vi "K2000_wait_get_array.vi"(2 "emergency exit":bool, 3 "samples":u64=4096, 4 "Readout parameters":T1(array[cluster])) -> (0 "requester status byte":i16, 1 "measures":sgl[][](array[numeric]))   [LabVIEW 2013]
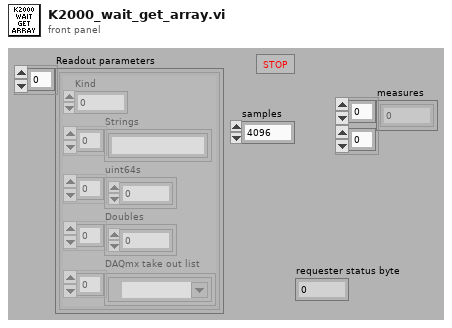
[diagram p1: front panel]
types:
  T1 = cluster{"Kind":u16, "Strings":string[], "uint64s":u64[], "Doubles":dbl[], "DAQmx take out list":refnum<k21>[]}[]
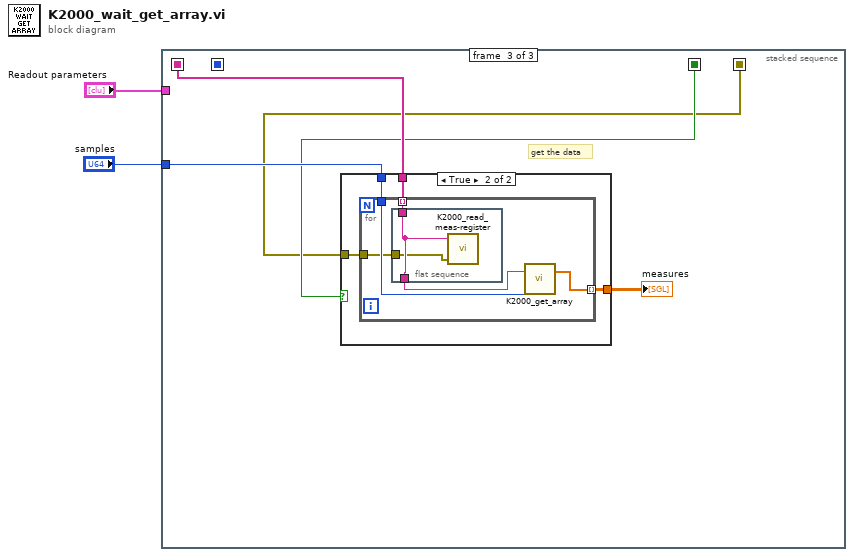
[diagram p0: block diagram]
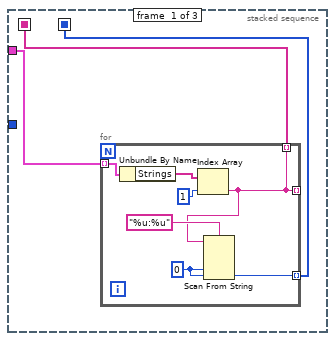
[diagram p2: hidden frame]
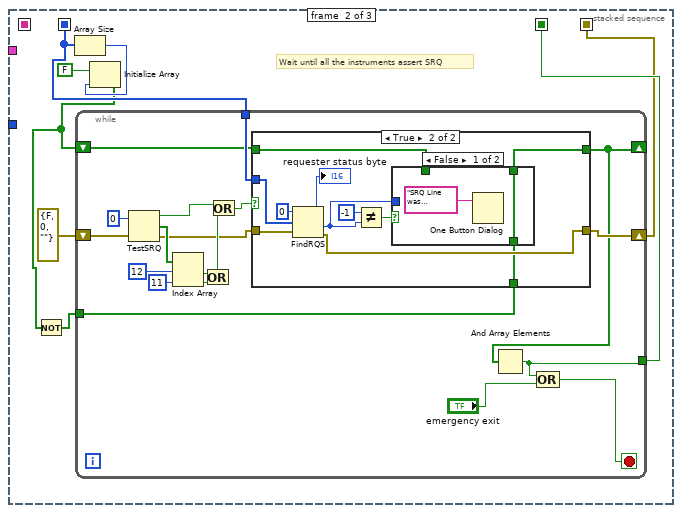
[diagram p3: hidden frame]
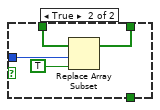
[diagram p5: hidden frame]
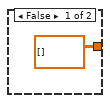
[diagram p6: hidden frame]
diagram:
  n1 = stacked-sequence {
    seq-local: [w4 _ _] -> [_ _ w62]
    seq-local: [w3 _ _] -> [_ w17 _]
    seq-local: [_ w14 _] -> [_ _ w60]
    seq-local: [_ w13 _] -> [_ _ w59]
    tunnel: "Readout parameters" -> [w5 _ _]
    tunnel: "samples" -> [_ _ w61]
    frame #0 {
      n2 = for {
        tunnel: w5 -> [w12] mode=indexing
        tunnel: [w6] -> _ mode=indexing
        tunnel: [w7] -> w3 mode=indexing
        tunnel: [w6] -> w4 mode=indexing
        w8 = u8 0
        n3 = Unbundle By Name(w12) -> ("Strings"=w11:string[])
        n4 = Index Array(array=w11, index=1) -> (element=w6:string)
        n5 = Scan From String(format string="%u:%u", input string=w6, default 1=w8, default 2=w8) -> (output 2=w7:u8)  [unwired: 3 in, 3 out]
      }
    }
    frame #1 {
      # "Wait until all the instruments assert SRQ"
      n6 = Array Size(array=w17) -> (size(s)=w18:i32)
      n7 = Initialize Array(FALSE ("Boolean"), w18) -> (w16:bool[])
      n8 = Not(x=w16) -> (.not. x?=w15:bool[])
      n9 = while {
        shift-right: [w24] -> _
        shift-left: w16 -> [w28]
        shift-right: [w25] -> w13
        shift-left: errorcluster {"status"=FALSE, "code"=0, "source"=""} ("error out") -> [w31]
        tunnel: w17 -> [w29]
        tunnel: w15 -> [w26]
        tunnel: [w21] -> w14
        stop <- w22 stop-if-true
        n10 = TestSRQ(0:0 ("bus"), 1:w31) -> (2:w32:bool, 3:w38:bool[], 4:w27:errorcluster)
        n11 = Index Array(array=w38, index #1=12 ("index"), index #2=11 ("index")) -> (element #1=w34:bool, element #2=w35:bool)
        n12 = Or(x=w34, y=w35) -> (x .or. y?=w33:bool)
        n13 = Or(x=w32, y=w33) -> (x .or. y?=w30:bool)
        n14 = case shown="True" w30 {
          tunnel: [w40 w51] -> w25
          tunnel: [w41 w47] -> w24
          tunnel: w27 -> [w40 w52]
          tunnel: w28 -> [w41 w46]
          tunnel: w29 -> [_ w49]
          tunnel: w26 -> [_ w42]
          frame False {
          }
          frame True {
            n15 = FindRQS(0:0 ("bus"), 1:w49, 2:w52) -> (3:→"requester status byte":i16, 5:w45:i32, 6:w51:errorcluster)  [unwired: 1 out]
            n16 = Not Equal?(x=-1, y=w45) -> (x != y?=w43:bool)
            n17 = case shown="False" w43 {
              tunnel: [w53 w58] -> w47
              tunnel: w46 -> [_ w57]
              tunnel: w45 -> [_ w56]
              tunnel: w42 -> [w53 _]
              frame False {
                n18 = One Button Dialog(message="SRQ Line was activated, but we couldn't\nfind the source of the SRQ.\nForcing the program to believe all the volmeters sent it...") -> ()  [unwired: 2 out]
              }
              frame True {
                n19 = Replace Array Subset(array=w57, new element=TRUE ("new element/subarray"), index=w56) -> (w58:bool[])
              }
            }
          }
        }
        n20 = And Array Elements(Boolean array=w24) -> (logical AND=w21:bool)
        n21 = Compound Arithmetic op=OR(w21, "emergency exit") -> (w22:bool)
      }
    }
    frame #2 {
      # "get the data"
      n22 = case shown="True" w60 {
        tunnel: [sgl[][] [] w66] -> w63
        tunnel: w61 -> [_ w68]
        tunnel: w62 -> [_ w67]
        tunnel: w59 -> [_ w65]
        frame False {
        }
        frame True {
          n23 = for {
            tunnel: w68 -> [w71]
            tunnel: w67 -> [w73] mode=indexing
            tunnel: [w70] -> w66 mode=indexing
            tunnel: w65 -> [w69]
            n24 = flat-sequence {
              tunnel: w73 -> [w75]
              tunnel: [w75] -> w72
              tunnel: w69 -> [w74]
              frame #0 {
                n25 = call "K2000_read_meas-register.vi"("error out 2"=w74, "GPIB Address"=w75) -> ()  [unwired: 3 out]
              }
            }
            n26 = call "K2000_get_array.vi"("samples"=w71, "address string"=w72) -> ("Array"=w70:sgl[])  [unwired: 1 out]
          }
        }
      }
      "measures" <- w63
    }
  }
